vi "Convert_Date_To_Time_Stamp.vi"(1 "Date (2016-12-31)":string="2016-12-31") -> (0 "Time Stamp en string":string)   [LabVIEW 2012]
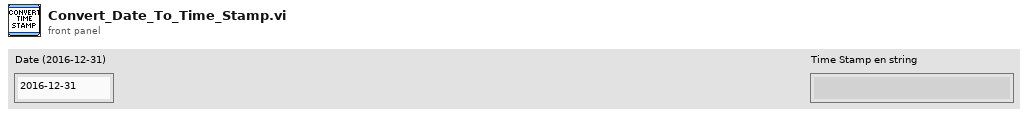
[diagram p1: front panel]
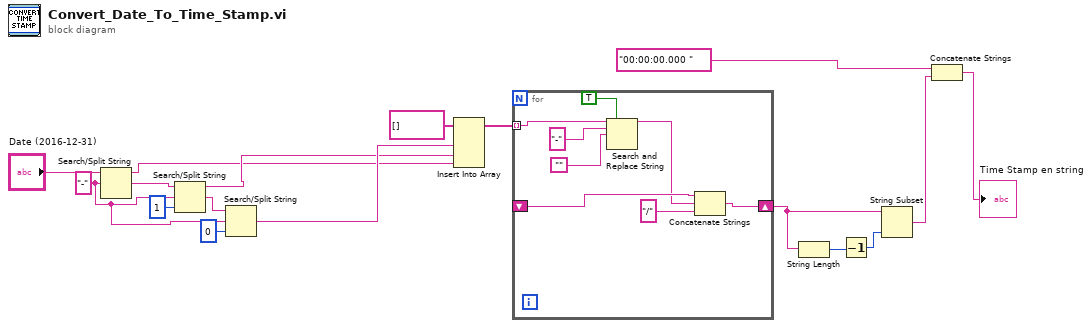
[diagram p0: block diagram]
diagram:
  w13 = "-" ("chaîne/car. recherché (-)")
  n1 = Search/Split String(string="Date (2016-12-31)", search string/char (-)=w13) -> (substring before match=w9:string, match + rest of string=w16:string)  [unwired: 1 in, 1 out]
  n2 = Search/Split String(string=w16, search string/char (-)=w13, offset (0)=1) -> (substring before match=w10:string, match + rest of string=w14:string)  [unwired: 1 out]
  n3 = Search/Split String(string=w14, search string/char (-)=w13, offset (0)=0) -> (match + rest of string=w11:string)  [unwired: 2 out]
  n4 = Insert Into Array(array=string[] [] ("tableau"), new element #1=w11, new element #2=w10, new element #3=w9) -> (w8:string[])  [unwired: 1 in]
  n5 = for {
    tunnel: w8 -> [w25] mode=indexing
    shift-right: [w20] -> w4
    shift-left: _ -> [w19]
    n6 = Search and Replace String(replace all?=TRUE ("tout remplacer ? (F)"), input string=w25, search string="-" ("chaîne recherchée"), replace string="") -> (result string=w18:string)  [unwired: 4 in, 3 out]
    n7 = Concatenate Strings(w19, w18, "/" ("chaîne")) -> (w20:string)
  }
  n8 = String Length(string=w4) -> (length=w6:i32)
  n9 = Decrement(x=w6) -> (x-1=w5:i32)
  n10 = String Subset(string=w4, length (rest)=w5) -> (substring=w2:string)  [unwired: 1 in]
  n11 = Concatenate Strings("00:00:00.000 ", w2) -> (→"Time Stamp en string":string)
